vi "Mq Sensor Labview.vi"() -> ()   [LabVIEW 2020]
uses:
  <vilib>/Instr/_visa.llb/VISA Configure Serial Port (Instr).vi
  <vilib>/Utility/file.llb/Write Delimited Spreadsheet (string).vi
panel:
  out "Digital Waveform Graph":T1(graph)
  in  "Table Control":string[][](table)
  in  "?":refnum<visa-resource-name>
  in  "?":bool
  in  "File Path":path
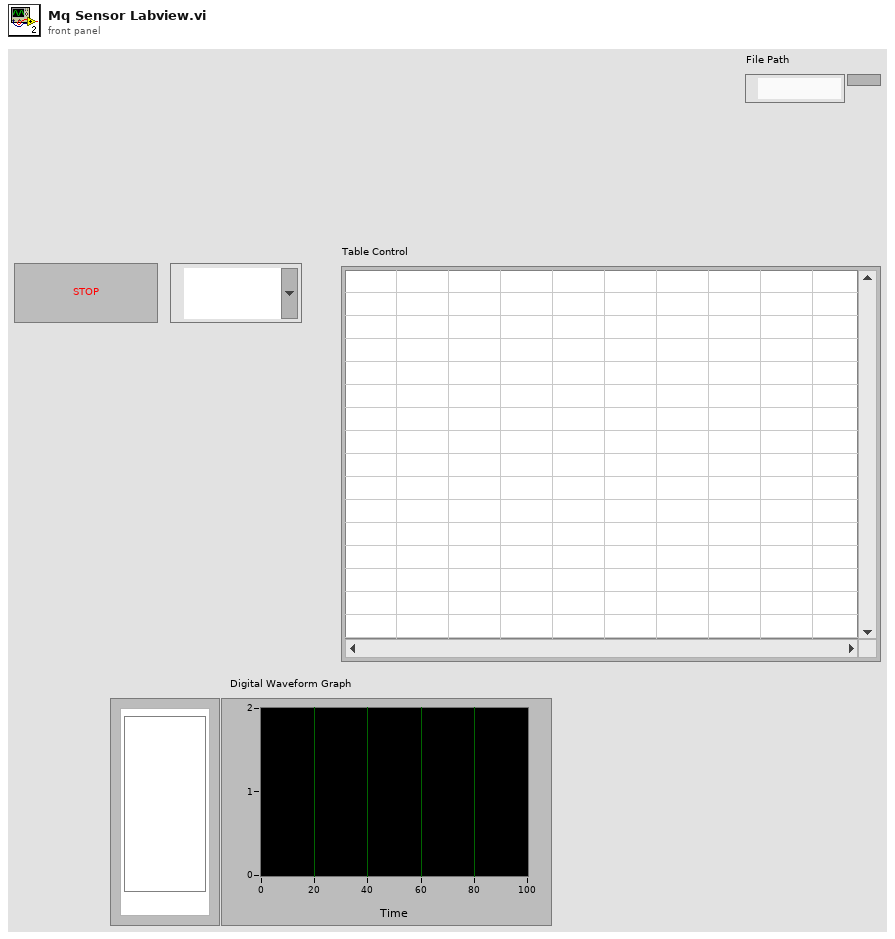
[diagram p1: front panel]
types:
  T1 = cluster{"x0":dbl, "dx":dbl, "[y]":u8[], "ports":i32}
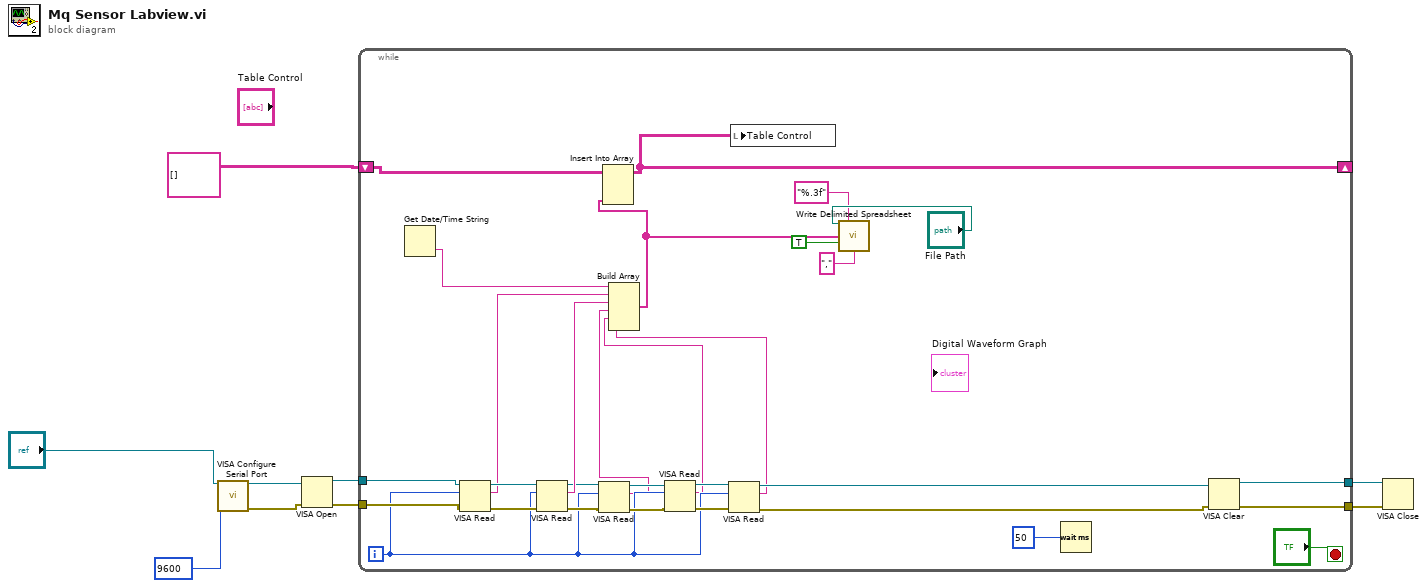
[diagram p0: block diagram]
diagram:
  n1 = call-poly "VISA Configure Serial Port"("VISA resource name"="?", "baud rate (9600)"=u32 9600) -> ("VISA resource name out"=w7:refnum<visa-resource-name>, "error out"=w6:errorcluster)  [unwired: 12 in]
  n2 = VISA Open(error in (no error)=w6, VISA resource name=w7) -> (VISA resource name=w5:refnum<visa-resource-name>, error out=w4:errorcluster)  [unwired: 3 in]
  n3 = while {
    tunnel: w5 -> [w38]
    tunnel: w4 -> [w37]
    tunnel: [w34] -> w3
    tunnel: [w33] -> w2
    shift-right: [w10] -> _
    shift-left: string[][] [] -> [w29]
    i -> [w15]
    stop <- "?" stop-if-true
    n4 = Get Date/Time String() -> (time string=w24:string)  [unwired: 3 in, 1 out]
    n5 = VISA Read(VISA resource name=w38, byte count=w15, error in (no error)=w37) -> (VISA resource name out=w36:refnum<visa-resource-name>, read buffer=w31:string, error out=w35:errorcluster)  [unwired: 1 out]
    n6 = VISA Read(VISA resource name=w36, byte count=w15, error in (no error)=w35) -> (VISA resource name out=w23:refnum<visa-resource-name>, read buffer=w30:string, error out=w19:errorcluster)  [unwired: 1 out]
    n7 = VISA Read(VISA resource name=w23, byte count=w15, error in (no error)=w19) -> (VISA resource name out=w22:refnum<visa-resource-name>, read buffer=w14:string, error out=w18:errorcluster)  [unwired: 1 out]
    n8 = VISA Read(VISA resource name=w22, byte count=w15, error in (no error)=w18) -> (VISA resource name out=w21:refnum<visa-resource-name>, read buffer=w13:string, error out=w17:errorcluster)  [unwired: 1 out]
    n9 = VISA Read(VISA resource name=w21, byte count=w15, error in (no error)=w17) -> (VISA resource name out=w20:refnum<visa-resource-name>, read buffer=w12:string, error out=w16:errorcluster)  [unwired: 1 out]
    n10 = Build Array(w24, w31, w30, w14, w13, w12) -> (w11:string[])
    n11 = Insert Into Array(array=w29, new element=w11) -> (w10:string[][])  [unwired: 2 in]
    n12 = local write "Table Control"(w10) -> ()
    n13 = call-poly <vilib>:"Write Delimited Spreadsheet.vi"("file path (dialog if empty)"="File Path", "format (%s)"="%.3f" ("format (%.3f)"), "1D data"=w11, "append to file? (new file:F)"=TRUE, "delimiter (\\t)"="," ("delimiter (\\t)")) -> ()  [unwired: 9 in, 2 out]
    n14 = Wait (ms)(milliseconds to wait=u32 50 ("millisecond timer value")) -> ()  [unwired: 1 out]
    n15 = VISA Clear(VISA resource name=w20, error in (no error)=w16) -> (VISA resource name out=w34:refnum<visa-resource-name>, error out=w33:errorcluster)
  }
  n16 = VISA Close(VISA resource name=w3, error in (no error)=w2) -> ()  [unwired: 1 out]
